vi "Example - Syslog Device.vi"() -> ()   [LabVIEW 2019, in "Logger.syslog.lvclass"]
doc: "This VI illustrates sending Syslog debug messages to a collector using the Syslog reference design library."
uses:
  Logger.syslog.lvclass
  <userlib>/_SEH/Controls/CEH/CEH Actions.ctl
  <vilib>/NI/syslog/_subVIs/TypeDefs/syslog_severity_codes.ctl
  <vilib>/NI/syslog/_subVIs/TypeDefs/syslog_facility_codes.ctl
  <userlib>/_OpenG.lib/numeric/numeric.llb/Random Number Within Range - DBL__ogtk.vi
panel:
  out "Syslog Messages Sent":string
  in  "Collector IP Address":string="0.0.0.0"
  in  "stop":bool
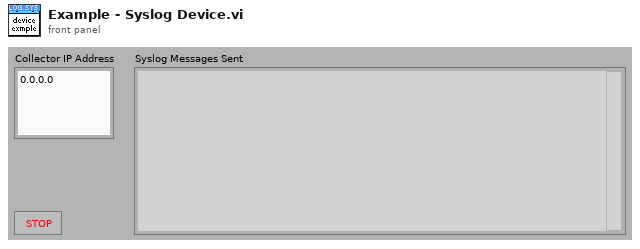
[diagram p1: front panel]
types:
  T1 = typedef "syslog_facility_codes.ctl" = enum16{"kernel", "user", "mail", "system daemons", "security/authorization", "syslogd", "line printer", "network news", "uucp", "clock daemon", "security/authorization (alternate)", "FTP daemon", "NTP subsystem", "log audit", "log alert", "clock daemon (alternate)", "local use 0", "local use 1", "local use 2", "local use 3", "local use 4", "local use 5", "local use 6", "local use 7"}
  T2 = typedef "syslog_severity_codes.ctl" = enum16{"emergency", "alert", "critical", "error", "warning", "notice", "info", "debug"}
  T3 = typedef "CEH Actions.ctl" = enum16{"Log", "Display Error Message", "Safe State", "Shutdown"}
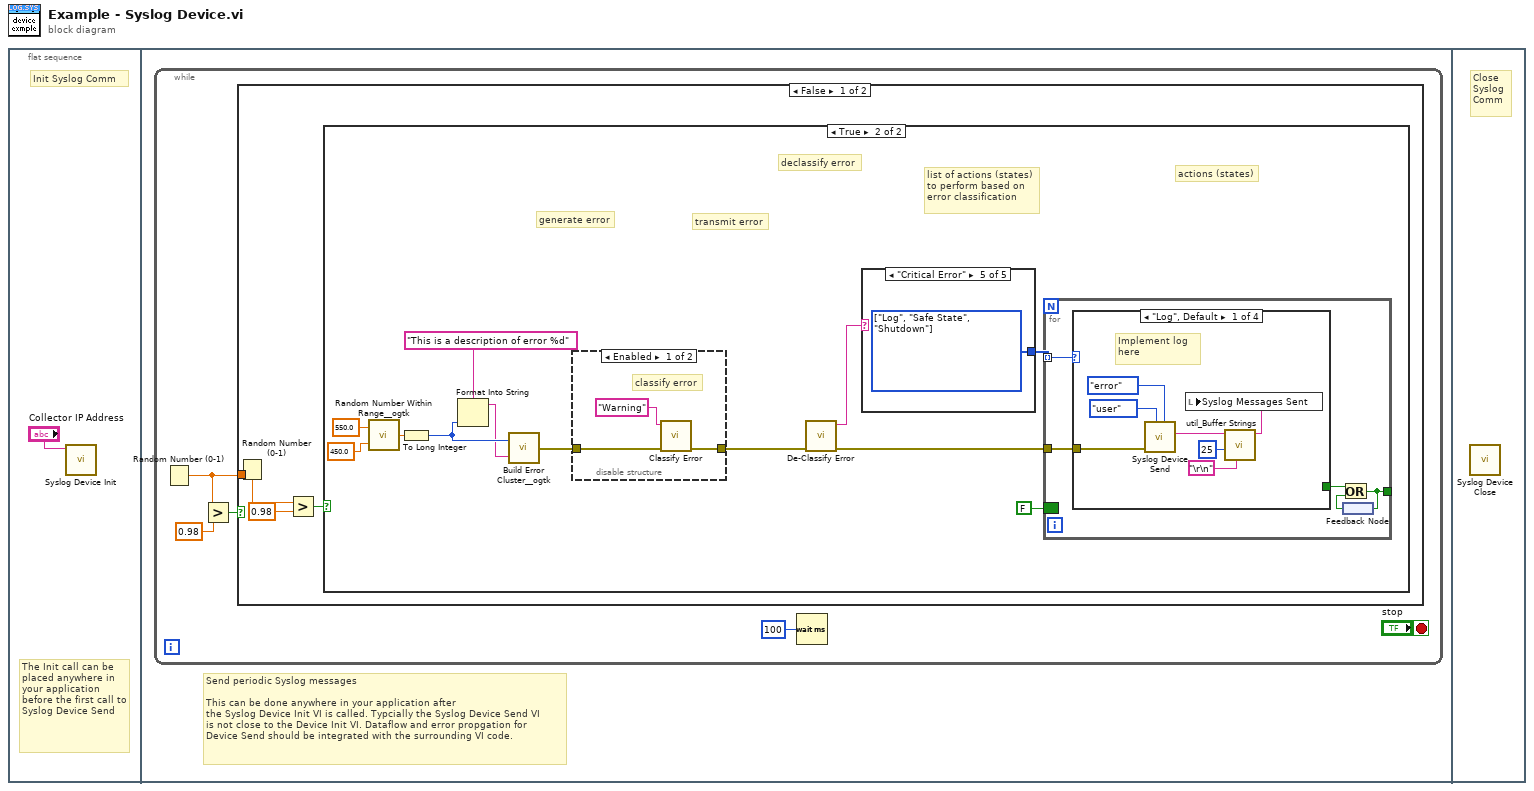
[diagram p0: block diagram]
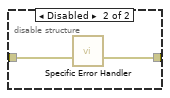
[diagram p3: hidden frame]
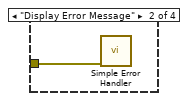
[diagram p4: hidden frame]
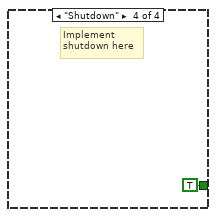
[diagram p6: hidden frame]
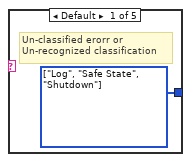
[diagram p7: hidden frame]
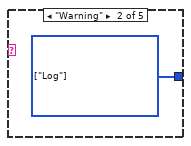
[diagram p8: hidden frame]
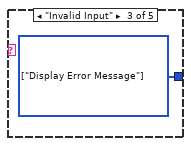
[diagram p9: hidden frame]
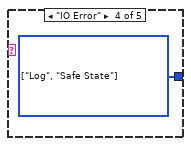
[diagram p10: hidden frame]
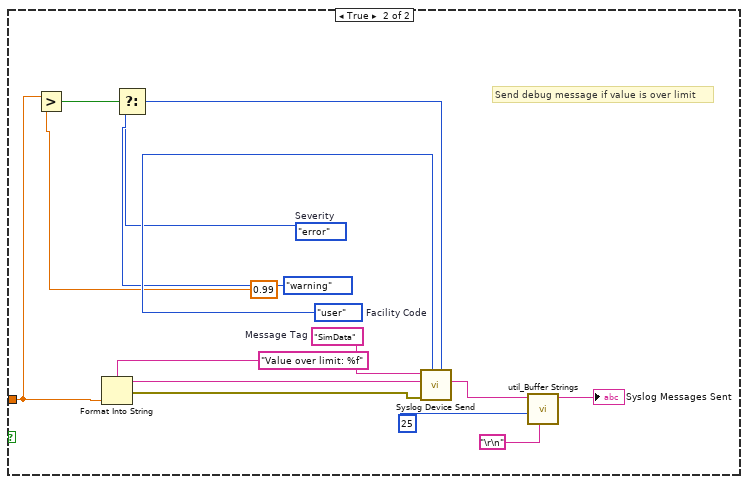
[diagram p11: hidden frame]
diagram:
  n1 = flat-sequence {
    frame #0 {
      # "The Init call can be placed anywhere in your application before the first call to Syslog Device Send"
      # "Init Syslog Comm"
      n2 = call <vilib>:"Syslog Device Init.vi"("Syslog Collector IP Address"="Collector IP Address") -> ()  [unwired: 10 in, 1 out]
    }
    frame #1 {
      # "Send periodic Syslog messages\n\nThis can be done anywhere in your application after\nthe Syslog Device Init VI is called. Typcially the Syslog Device Send VI\nis not close to the Device Init VI. Dataflow and error propgation for \nDevice Send should be integrated with the surrounding VI code."
      n3 = while {
        stop <- "stop" stop-if-true
        n4 = Random Number (0-1)() -> (number: 0 to 1=w2:dbl)
        n5 = Greater?(x=w2, y=0.98) -> (0:w3:bool)
        n6 = case shown="False" w3 {
          tunnel: w2 -> [_ w57]
          frame False {
            n7 = Random Number (0-1)() -> (number: 0 to 1=w9:dbl)
            n8 = Greater?(x=w9, y=0.98) -> (0:w7:bool)
            n9 = case shown="True" w7 {
              frame False {
              }
              frame True {
                # "actions (states)"
                # "list of actions (states)\nto perform based on\nerror classification"
                # "declassify error"
                # "transmit error"
                # "generate error"
                n10 = call-poly <userlib>:"Random Number Within Range__ogtk.vi"("High"=550.0, "Low"=450.0) -> ("Random Number"=w19:dbl)  [unwired: 3 in]
                n11 = To Long Integer(number=w19) -> (32bit integer=w18:i32)
                n12 = Format Into String(format string="This is a description of error %d" ("String to Prepend to source (\"\")"), w18) -> (resulting string=w10:string)  [unwired: 2 in, 1 out]
                n13 = call <userlib>:"Build Error Cluster__ogtk.vi"("String to Prepend to source (\"\")"=w10, "code"=w18) -> ("error out"=w11:errorcluster)
                n14 = disable-structure shown="Enabled" {
                  disable-tunnel: [w24 w25] -> w16
                  disable-tunnel: w11 -> [w23 w26]
                  frame Enabled {
                    # "classify error"
                    n15 = call <userlib>:"Classify Error.vi"("Error to Classify"=w23, "String"="Warning") -> ("Classified Error"=w24:errorcluster)  [unwired: 9 in]
                  }
                  frame Disabled {
                    n16 = call "Specific Error Handler"("Error to Check"=w26) -> ("error out"=w25:errorcluster)  [unwired: 11 in, 3 out]
                  }
                }
                n17 = call <userlib>:"De-Classify Error.vi"("Classified Error"=w16) -> ("De-Classified Error"=w14:errorcluster, "Error Classification"=w13:string)  [unwired: 8 in, 1 out]
                n18 = case shown="\"Critical Error\"" w13 {
                  tunnel: [w41 w42 w43 w44 w45] -> w15
                  frame Default {
                    w41 = T3[] [enum."Log", enum."Safe State", enum."Shutdown"] items=["Log", "Display Error Message", "Safe State", "Shutdown"]
                    # "Un-classified erorr or\nUn-recognized classification"
                  }
                  frame "Warning" {
                    w42 = T3[] [enum."Log"] items=["Log", "Display Error Message", "Safe State", "Shutdown"]
                  }
                  frame "Invalid Input" {
                    w43 = T3[] [enum."Display Error Message"] items=["Log", "Display Error Message", "Safe State", "Shutdown"]
                  }
                  frame "IO Error" {
                    w44 = T3[] [enum."Log", enum."Safe State"] items=["Log", "Display Error Message", "Safe State", "Shutdown"]
                  }
                  frame "Critical Error" {
                    w45 = T3[] [enum."Log", enum."Safe State", enum."Shutdown"] items=["Log", "Display Error Message", "Safe State", "Shutdown"]
                  }
                }
                n19 = for {
                  tunnel: w14 -> [w30]
                  tunnel: w15 -> [w31] mode=indexing
                  border: FALSE -> [_]
                  tunnel: [w27] -> _
                  n20 = case shown="\"Log\", Default" w31 {
                    tunnel: w30 -> [w37 w39 _ _]
                    tunnel: [_ _ _ TRUE] -> w29
                    frame "Log", Default {
                      # "Implement log \nhere"
                      n21 = call <vilib>:"Syslog Device Send.vi"("Severity Code (error)"=syslog_severity_codes."error", "Facility Code (user)"=syslog_facility_codes."user", "error in (no error)"=w37) -> ("Syslog Message"=w33:string)  [unwired: 7 in, 1 out]
                      n22 = call <vilib>:"util_Buffer Strings.vi"("Insert between Strings (\"\")"="\r\n", "Number of Strings to Buffer"=u8 25, "New String"=w33) -> ("Buffered String Series"=w32:string)  [unwired: 8 in]
                      n23 = local write "Syslog Messages Sent"(w32) -> ()
                    }
                    frame "Display Error Message" {
                      n24 = call <vilib>:"Simple Error Handler.vi"("error in (no error)"=w39) -> ()  [unwired: 4 in, 5 out]
                    }
                    frame "Safe State" {
                      # "Implement safe\nstate here"
                    }
                    frame "Shutdown" {
                      # "Implement\nshutdown here"
                    }
                  }
                  n25 = feedback #1() -> (w28:bool)
                  n26 = Or(x=w29, y=w28) -> (x .or. y?=w27:bool)
                  n27 = feedback-in #1(w27) -> ()
                }
              }
            }
          }
          frame True {
            w47 = "SimData"  # Message Tag
            w54 = syslog_severity_codes."error"  # Severity
            w60 = syslog_facility_codes."user"  # Facility Code
            # "Send debug message if value is over limit"
            n28 = Greater?(x=w57, y=0.99) -> (0:w56:bool)
            n29 = Format Into String(format string="Value over limit: %f", w57) -> (resulting string=w49:string, error out=w52:errorcluster)  [unwired: 2 in]
            n30 = Select(t=w54, s=w56, f=syslog_severity_codes."warning" ("Severity (error)")) -> (s? t:f=w53:T2)
            n31 = call <vilib>:"Syslog Device Send.vi"("Severity Code (error)"=w53, "Facility Code (user)"=w60, "error in (no error)"=w52, "Message Content"=w49, "Message Tag"=w47) -> ("Syslog Message"=w48:string)  [unwired: 5 in, 1 out]
            n32 = call <vilib>:"util_Buffer Strings.vi"("Insert between Strings (\"\")"="\r\n", "Number of Strings to Buffer"=u8 25, "New String"=w48) -> ("Buffered String Series"=→"Syslog Messages Sent":string)  [unwired: 8 in]
          }
        }
        n33 = Wait (ms)(milliseconds to wait=u32 100 ("millisecond multiple")) -> ()  [unwired: 1 out]
      }
    }
    frame #2 {
      # "Close\nSyslog\nComm"
      n34 = call <vilib>:"Syslog Device Close.vi"() -> ()  [unwired: 11 in, 1 out]
    }
  }
